vi "update_indicators.vi"(9 "New length":dbl, 10 "Neuron number":u16, 11 "Control references":T1) -> (3 "score":dbl)   [LabVIEW 2011]
uses:
  typedefs/control_references_cluster.ctl
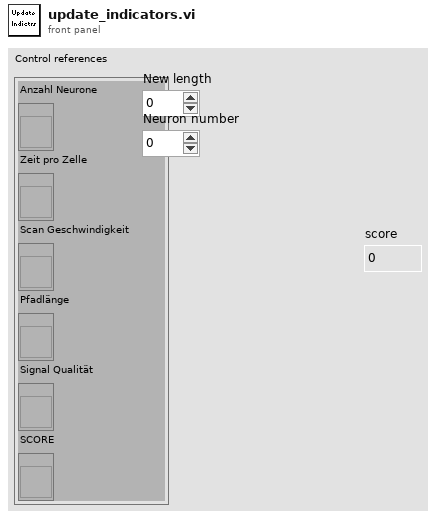
[diagram p1: front panel]
types:
  T1 = typedef "control_references_cluster.ctl" = cluster{"Anzahl Neurone":refnum<vi>, "Zeit pro Zelle":refnum<vi>, "Scan Geschwindigkeit":refnum<vi>, "Pfadlänge":refnum<vi>, "Signal Qualität":refnum<vi>, "SCORE":refnum<vi>}
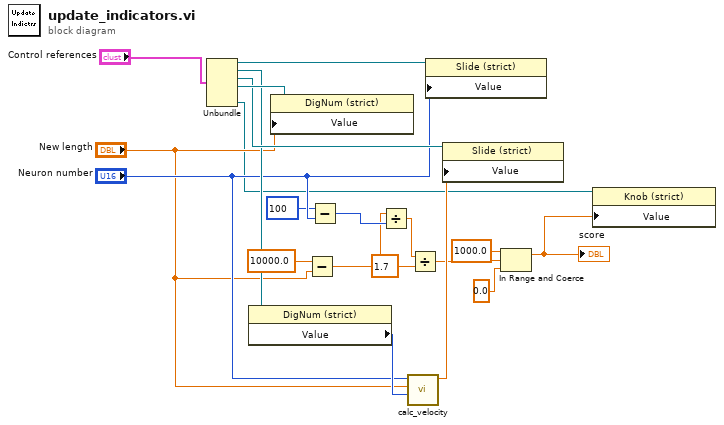
[diagram p0: block diagram]
diagram:
  n1 = Unbundle("Control references") -> ("Anzahl Neurone"=w18:refnum<vi>, "Zeit pro Zelle"=w16:refnum<vi>, "Scan Geschwindigkeit"=w17:refnum<vi>, "Pfadlänge"=w19:refnum<vi>, "SCORE"=w2:refnum<vi>)  [unwired: 1 out]
  n2 = property class="DigNum (strict)"(reference=w16) -> ("Value"=w14:i32)  [unwired: 1 in, 2 out]
  n3 = property class="DigNum (strict)"(reference=w19, "Value"="New length") -> ()  [unwired: 1 in, 2 out]
  n4 = Subtract(x=10000.0, y="New length") -> (x-y=w8:dbl)
  n5 = Subtract(x=u16 100 ("y"), y="Neuron number") -> (x-y=w11:u16)
  n6 = Divide(x=w8, y=w11) -> (x/y=w7:dbl)
  n7 = call "calc_velocity.vi"("Time per cell"=w14, "Path length"="New length", "Neurons"="Neuron number") -> ("Velocity"=w15:dbl)  [unwired: 8 in]
  n8 = Divide(x=w7, y=1.7) -> (x/y=w5:dbl)
  n9 = property class="Slide (strict)"(reference=w18, "Value"="Neuron number") -> ()  [unwired: 1 in, 2 out]
  n10 = property class="Slide (strict)"(reference=w17, "Value"=w15) -> ()  [unwired: 1 in, 2 out]
  n11 = In Range and Coerce(upper limit=1000.0, x=w5, lower limit=0.0) -> (coerced(x)=w1:dbl)  [unwired: 1 out]
  "score" <- w1
  n12 = property class="Knob (strict)"(reference=w2, "Value"=w1) -> ()  [unwired: 1 in, 2 out]
